vi "Exp no 6b Application Using FOR LOOP.vi"() -> ()   [LabVIEW 2010]
panel:
  out "Sum of N^2 Numbers":i32[](array[numeric])
  in  "N":i32
  # "SUM OF N^2 NUMBERS"
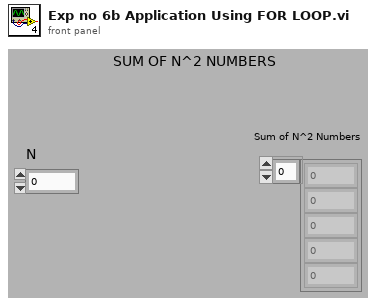
[diagram p1: front panel]
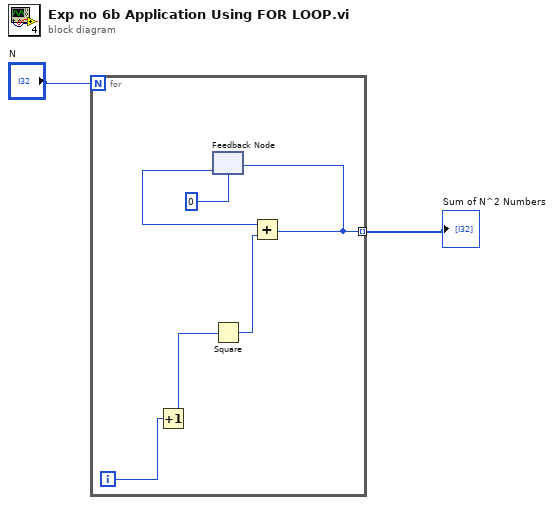
[diagram p0: block diagram]
diagram:
  n1 = for {
    N: "N" -> [_]
    tunnel: [w4] -> w2 mode=indexing
    i -> [w8]
    n2 = Increment(x=w8) -> (x+1=w7:i32)
    n3 = feedback #1(0) -> (w3:i32)
    n4 = Square(x=w7) -> (x^2=w6:i32)
    n5 = Add(x=w3, y=w6) -> (x+y=w4:i32)
    n6 = feedback-in #1(w4) -> ()
  }
  "Sum of N^2 Numbers" <- w2
